vi "TCP Vision - Receiver.vi"(10 "receiver port":u16=1180) -> (2 "Image":T1(plugin-control))   [LabVIEW 2023]
doc: "The UDP protocol differs from TCP in that there is no error-checking with the packets of information that are sent, and thus no guarantee whatsoever that an intended recipient will actually receive a given piece of data.\n\nUDP does offer the ability to \"broadcast\" data across a network--simply specify an IP Address of all ones (255.255.255.255) to attempt to broadcast information network-wide. Keep in mind that routers and other network hardware will generally refuse to forward the broadcast beyond certain points, so the extent of the broadcast will in practice be limited."
uses:
  Vision Server/TCP Main States.ctl
  <vilib>/vision/Image Controls.llb/IMAQ Image.ctl
  <vilib>/Rock Robotics/Network Tables/NT Read String.vi
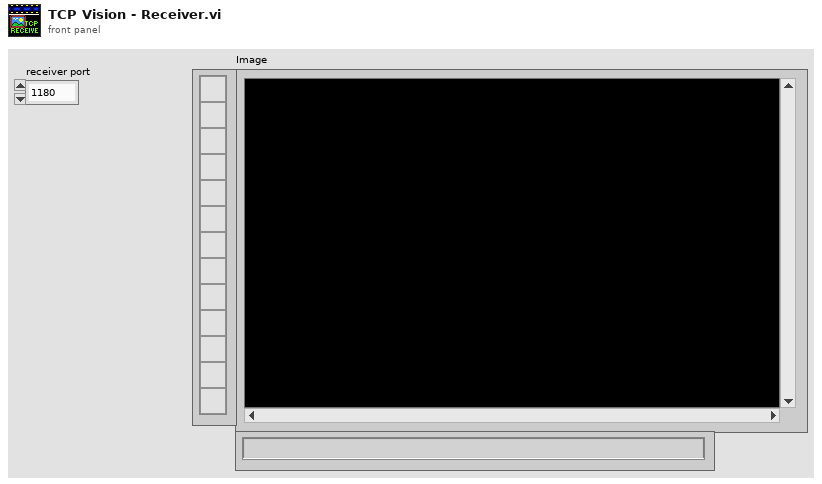
[diagram p1: front panel]
types:
  T1 = typedef "IMAQ Image.ctl" = refnum<image>
  T2 = typedef "TCP Main States.ctl" = enum16{"Message Dispatcher", "INI", "Read Data", "Send Data", "TCP Close", "TCP Open", "Exit"}
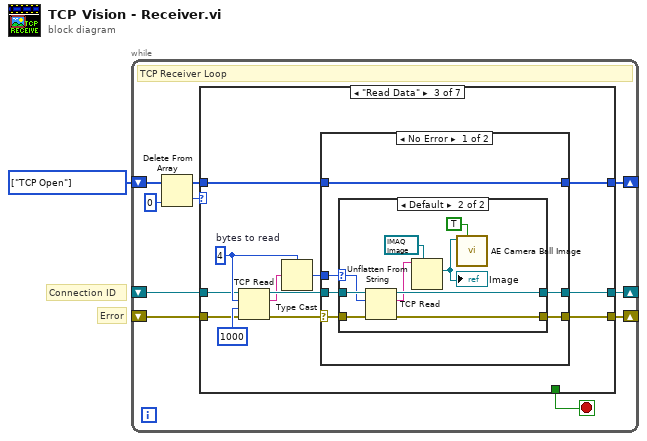
[diagram p0: block diagram]
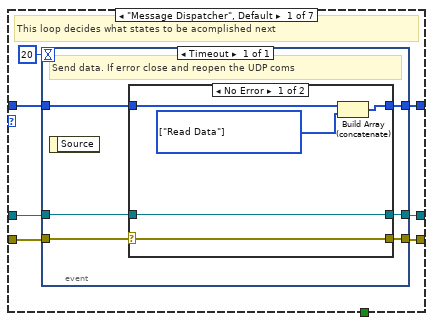
[diagram p2: hidden frame]
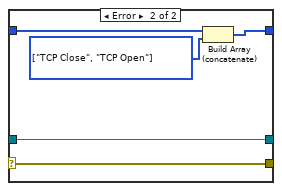
[diagram p3: hidden frame]
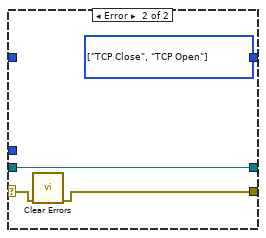
[diagram p6: hidden frame]
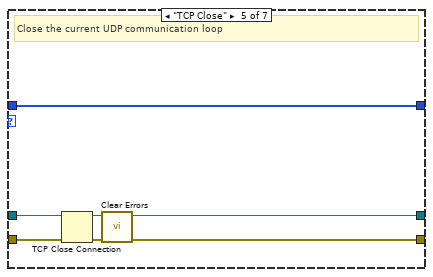
[diagram p8: hidden frame]
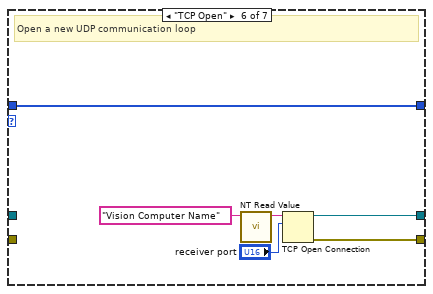
[diagram p9: hidden frame]
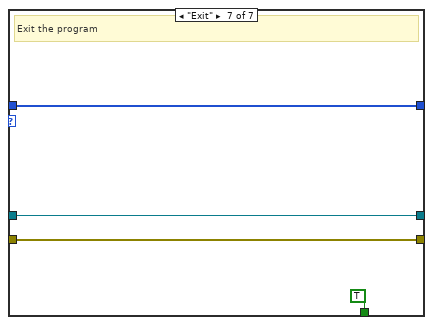
[diagram p10: hidden frame]
diagram:
  w1 = T2[] [enum."TCP Open"] items=["Message Dispatcher", "INI", "Read Data", "Send Data", "TCP Close", "TCP Open", "Exit"]
  # "Error"
  # "Connection ID"
  n1 = while {
    shift-right: [w3] -> _
    shift-left: w1 -> [w7]
    shift-right: [w11] -> _
    shift-left: _ -> [w9]
    shift-right: [w10] -> _
    shift-left: _ -> [w8]
    stop <- w2 stop-if-true
    # "TCP Receiver Loop"
    n2 = Delete From Array(array=w7, index=0) -> (deleted portion=w5:T2, array with subset deleted=w4:T2[])  [unwired: 1 in]
    n3 = case shown="\"Read Data\"" w5 {
      tunnel: [w15 w37 w42 w72 w74 w83 w89] -> w11
      tunnel: [w13 w36 w41 w71 w75 w82 w88] -> w10
      tunnel: w9 -> [w16 w37 w44 w72 w78 _ w89]
      tunnel: w8 -> [w14 w36 w43 w71 w77 _ w88]
      tunnel: w4 -> [w18 w35 w39 w73 w79 w85 w87]
      tunnel: [w17 w35 w38 w73 w79 w85 w87] -> w3
      tunnel: [_ _ _ _ _ _ TRUE] -> w2
      frame "Message Dispatcher", Default {
        # "This loop decides what states to be acomplished next"
        n4 = event shown="[0] Timeout" {
          selector: _ -> [_]
          dyn-events: _ -> [_]
          timeout: 20 -> [_]
          tunnel: w18 -> [w22]
          tunnel: [w21] -> w17
          tunnel: w16 -> [w20]
          tunnel: [w19] -> w15
          tunnel: w14 -> [w24]
          tunnel: [w23] -> w13
          event Timeout {
            # "Send data. If error close and reopen the UDP coms"
            n5 = event-data() -> ()  [unwired: 1 in, 1 out]
            n6 = case shown="No Error" w24 {
              selector: w24 -> [w29 w34]
              tunnel: [w29 w34] -> w23
              tunnel: w22 -> [w28 w33]
              tunnel: [w26 w31] -> w21
              tunnel: w20 -> [w27 w32]
              tunnel: [w27 w32] -> w19
              frame No Error {
                w25 = T2[] [enum."Read Data"] items=["Message Dispatcher", "INI", "Read Data", "Send Data", "TCP Close", "TCP Open", "Exit"]
                n7 = Build Array (concatenate)(w28, w25) -> (w26:T2[])
              }
              frame Error {
                w30 = T2[] [enum."TCP Close", enum."TCP Open"] items=["Message Dispatcher", "INI", "Read Data", "Send Data", "TCP Close", "TCP Open", "Exit"]
                n8 = Build Array (concatenate)(w33, w30) -> (w31:T2[])
              }
            }
          }
        }
      }
      frame "INI" {
      }
      frame "Read Data" {
        w45 = 4  # bytes to read
        n9 = TCP Read(connection ID=w44, bytes to read=w45, error in (no error)=w43, 9:1000 ("timeout ms (25000)")) -> (connection ID out=w48:refnum<k5>, data out=w47:string, error out=w40:errorcluster)  [unwired: 1 in]
        n10 = Type Cast(type=w45, x=w47) -> (*(type *) &x=w49:i32)
        n11 = case shown="No Error" w40 {
          selector: w40 -> [w51 w69]
          tunnel: w49 -> [w55 _]
          tunnel: w48 -> [w54 w68]
          tunnel: [w53 w68] -> w42
          tunnel: [w52 w67] -> w41
          tunnel: w39 -> [w50 _]
          tunnel: [w50 w70] -> w38
          frame No Error {
            n12 = case shown="Default" w55 {
              selector: w55 -> [_ w62]
              tunnel: w54 -> [w57 w66]
              tunnel: w51 -> [w56 w65]
              tunnel: [w57 w64] -> w53
              tunnel: [w56 w63] -> w52
              frame ..0 {
                # "The server has not written any data"
              }
              frame Default {
                n13 = TCP Read(connection ID=w66, bytes to read=w62, error in (no error)=w65) -> (connection ID out=w64:refnum<k5>, data out=w58:string, error out=w63:errorcluster)  [unwired: 2 in]
                n14 = Unflatten From String(type=T1 refnum ("Image"), binary string=w58) -> (value=w60:T1)  [unwired: 3 in, 2 out]
                "Image" <- w60
                n15 = call "AE Camera Ball Image.vi"("Update"=TRUE, "Ball Image in"=w60) -> ()  [unwired: 9 in, 1 out]
              }
            }
          }
          frame Error {
            w70 = T2[] [enum."TCP Close", enum."TCP Open"] items=["Message Dispatcher", "INI", "Read Data", "Send Data", "TCP Close", "TCP Open", "Exit"]
            n16 = call <vilib>:"Clear Errors.vi"("error in (no error)"=w69) -> ("error out"=w67:errorcluster)  [unwired: 5 in, 1 out]
          }
        }
      }
      frame "Send Data" {
        # "Sends camera images to the dashboard"
      }
      frame "TCP Close" {
        # "Close the current UDP communication loop"
        n17 = TCP Close Connection(connection ID=w78, error in (no error)=w77) -> (connection ID out=w74:refnum<k5>, error out=w76:errorcluster)  [unwired: 1 in]
        n18 = call <vilib>:"Clear Errors.vi"("error in (no error)"=w76) -> ("error out"=w75:errorcluster)  [unwired: 5 in, 1 out]
      }
      frame "TCP Open" {
        # "Open a new UDP communication loop"
        n19 = call-poly <vilib>:"NT Read Value.vi"("name"="Vision Computer Name" ("Name")) -> ("value"=w80:string)  [unwired: 8 in, 2 out]
        n20 = TCP Open Connection(address=w80, remote port or service name="receiver port") -> (connection ID=w83:refnum<k5>, error out=w82:errorcluster)  [unwired: 3 in]
      }
      frame "Exit" {
        # "Exit the program"
      }
    }
  }
